vi "Get Connection Description Text and Pins Tab.vi"(11 "Mode":T2) -> (2 "Pins tab":T1, 3 "Description":string)   [LabVIEW 2019, in "NI Synchronization System Explorer.lvlib"]
uses:
  NI Synchronization System Explorer.lvlib
  Shared/Mode.ctl
  Pins Tab.ctl
  Shared/Constants.vi
  Shared/NI Synchronization Shared.lvlib
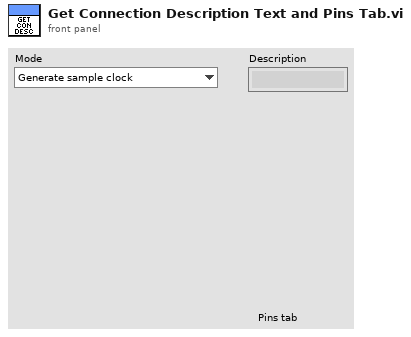
[diagram p1: front panel]
types:
  T1 = typedef "NI Synchronization System Explorer.lvlib/Pins Tab.ctl" = enum32{"Pins", "Ext. Pin", "Custom"}
  T2 = typedef "NI Synchronization Shared.lvlib/Mode.ctl" = enum16{"Generate sample clock", "Route sample clock out of chassis", "Route sample clock into chassis", "Custom routes"}
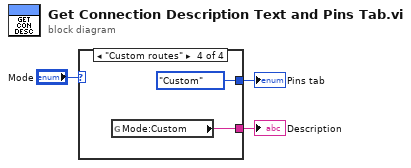
[diagram p0: block diagram]
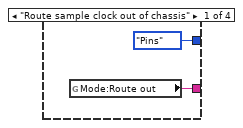
[diagram p2: hidden frame]
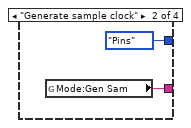
[diagram p3: hidden frame]
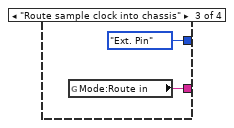
[diagram p4: hidden frame]
diagram:
  n1 = case shown="\"Custom routes\"" "Mode" {
    tunnel: [w5 w7 w9 w10] -> w3
    tunnel: [Pins_Tab."Pins" ("Pins tab") Pins_Tab."Pins" ("Pins tab") Pins_Tab."Ext. Pin" ("Pins tab") Pins_Tab."Custom" ("Pins tab")] -> w1
    frame "Route sample clock out of chassis" {
      n2 = global read "Constants.vi" "Mode:Route out"() -> (w5:string)
    }
    frame "Generate sample clock" {
      n3 = global read "Constants.vi" "Mode:Gen Sam"() -> (w7:string)
    }
    frame "Route sample clock into chassis" {
      n4 = global read "Constants.vi" "Mode:Route in"() -> (w9:string)
    }
    frame "Custom routes" {
      n5 = global read "Constants.vi" "Mode:Custom"() -> (w10:string)
    }
  }
  "Description" <- w3
  "Pins tab" <- w1
